vi "ShowWavSpectrum.vi"() -> ()   [LabVIEW 2013]
doc: "This is demo for wav sound file specturem viewer."
uses:
  <vilib>/sound2/lvsound2.llb/Sound File Read (DBL).vi
  <vilib>/sound2/lvsound2.llb/Sound File Read Open.vi
  <vilib>/measure/NI_MAPro.lvlib
  <vilib>/sound2/lvsound2.llb/Sound File Position.ctl
  <vilib>/measure/maspectr.llb/FFT Spectrum (Mag-Phase) for 1 Chan.vi
  <vilib>/Waveform/WDTOps.llb/WDT Get Waveform Subset DBL.vi
panel:
  in  "Stop Button":bool
  in  "Duration":dbl=100.0
  in  "Tunnel":i32
  in  "File Path Control":path
  out "SoundBar":cluster{dbl[], dbl[]}(graph)
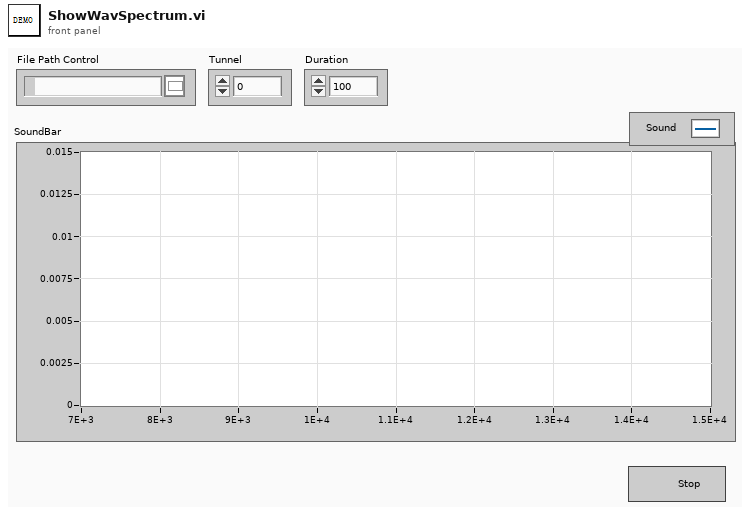
[diagram p1: front panel]
types:
  T1 = typedef "Sound File Position.ctl" = u16
  T2 = typedef "Sound File Refnum.ctl" = refnum<file>
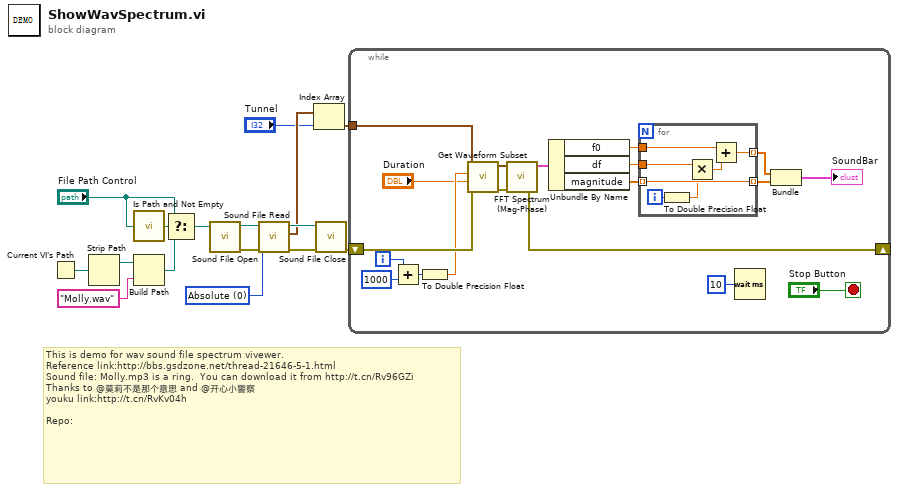
[diagram p0: block diagram]
diagram:
  w14 = T1 0 items=["Absolute"=0, "Relative"=2] ("position mode")
  # "This is demo for wav sound file spectrum vivewer.\nReference link:http://bbs.gsdzone.net/thread-21646-5-1.html\nSound file: Molly.mp3 is a ring.  You can download it from http://t.cn/Rv96GZi\nThanks to @莫莉不是那个意思 and @开心小警察\nyouku link:http://t.cn/RvKv04h\n\nRepo:"
  n1 = Current VI's Path() -> (path=w8:path)
  n2 = Strip Path(path=w8) -> (stripped path=w7:path)  [unwired: 1 out]
  n3 = call <vilib>:"Is Path and Not Empty.vi"("path"="File Path Control") -> ("Is Path and Not Empty?"=w5:bool)  [unwired: 4 in]
  n4 = Build Path(base path=w7, name or relative path="Molly.wav") -> (appended path=w3:path)
  n5 = Select(t="File Path Control", s=w5, f=w3) -> (s? t:f=w2:path)
  n6 = call-poly <vilib>:"Sound File Open.vi"("path"=w2) -> ("error out"=w11:errorcluster, "sound file refnum"=w16:T2)  [unwired: 9 in]
  n7 = call-poly <vilib>:"Sound File Read.vi"("error in (no error)"=w11, "position mode"=w14, "sound file refnum"=w16) -> ("error out"=w10:errorcluster, "data"=w13:waveform(dbl)[], "sound file refnum out"=w15:T2)  [unwired: 4 in, 2 out]
  n8 = Index Array(array=w13, index="Tunnel") -> (element=w12:waveform(dbl))
  n9 = call <vilib>:"Sound File Close.vi"("error in (no error)"=w10, "sound file refnum"=w15) -> ("error out"=w9:errorcluster)  [unwired: 9 in]
  n10 = while {
    tunnel: w12 -> [w30]
    shift-right: [w25] -> _
    shift-left: w9 -> [w26]
    i -> [w19]
    stop <- "Stop Button" stop-if-true
    n11 = Add(x=w19, y=1000) -> (x+y=w17:i32)
    n12 = To Double Precision Float(number=w17) -> (double precision float=w23:dbl)
    n13 = call-poly <vilib>:"Get Waveform Subset.vi"("error in (no error)"=w26, "duration"="Duration", "start samples/time"=w23, "waveform in"=w30) -> ("error out"=w27:errorcluster, "waveform out"=w29:waveform(dbl))  [unwired: 2 in, 2 out]
    n14 = call-poly <vilib>:"FFT Spectrum (Mag-Phase).vi"("error in (no error)"=w27, "time signal"=w29) -> ("error out"=w25:errorcluster, "magnitude"=w22:cluster{"f0":dbl, "df":dbl, "magnitude":dbl[]})  [unwired: 5 in, 3 out]
    n15 = Unbundle By Name(w22) -> ("f0"=w34:dbl, "df"=w33:dbl, "magnitude"=w35:dbl[])
    n16 = for {
      tunnel: w35 -> [w38] mode=indexing
      tunnel: w34 -> [w41]
      tunnel: w33 -> [w42]
      tunnel: [w39] -> w32 mode=indexing
      tunnel: [w38] -> w31 mode=indexing
      i -> [w37]
      n17 = To Double Precision Float(number=w37) -> (double precision float=w36:dbl)
      n18 = Multiply(x=w42, y=w36) -> (x*y=w40:dbl)
      n19 = Add(x=w41, y=w40) -> (x+y=w39:dbl)
    }
    n20 = Wait (ms)(milliseconds to wait=u32 10) -> ()  [unwired: 1 out]
    n21 = Bundle(w32, w31) -> (→"SoundBar":cluster{dbl[], dbl[]})  [unwired: 1 in]
  }
